vi "Multiple ToFs.vi"() -> ()   [LabVIEW 2014]
uses:
  <vilib>/Analysis/baseanly.llb/Mean (DBL).vi
  <vilib>/MakerHub/LINX/Public/Utilities/Open Local.vi
  <vilib>/MakerHub/LINX/LMH-LINX.lvlib
  <vilib>/Analysis/NI_AALBase.lvlib
panel:
  out "Sensor Error Code":u8
  out "Attempts":i32
  out "ToF 4":u8(slide) scale=0.0..80.0
  out "ToF 3":u8(slide) scale=0.0..80.0
  out "ToF 2":u8(slide) scale=0.0..80.0
  out "ToF 1":u8(slide) scale=0.0..80.0
  out "error out":errorcluster
  in  "Speed Read":bool
  out "Loop Rate (Hz)":u32
  out "range":dbl
  out "Array":dbl[](array[numeric])
  out "min value":dbl
  out "max value":dbl
  in  "Samples to Avg":i32=10
  in  "milliseconds to wait":u32=20
  in  "Stop":bool
  out "Distance":cluster{"Distance (mm)":u8, u8}(graph)
  # "0 = No error\n6 = early convergence estimate check failed\n7 = max convergence issue"
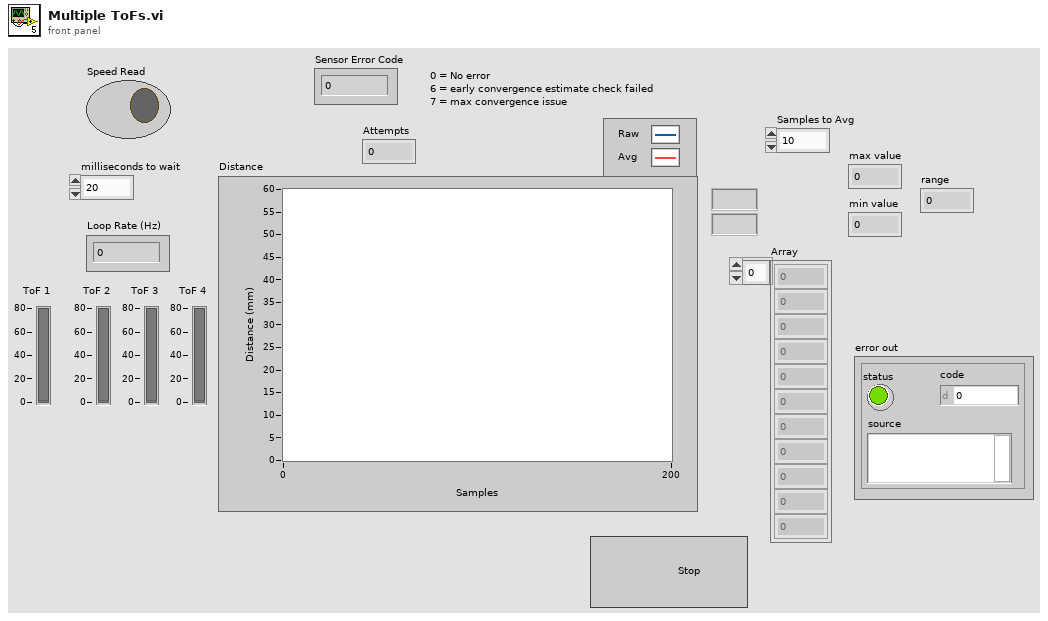
[diagram p1: front panel]
types:
  T1 = typedef "LMH-LINX.lvlib/LINX Ref.ctl" = cluster{"IO":T2, "Interface":T3, "LINX Device Config":T4}
  T2 = typedef "LMH-LINX.lvlib/Platform.ctl" = enum16{"Remote", "Local"}
  T3 = typedef "LMH-LINX.lvlib/Interface.ctl" = enum16{"Serial", "TCP"}
  T4 = typedef "LMH-LINX.lvlib/Device.lvlib/LINX Device Config.ctl" = cluster{"Interface":T3, "COM Port":refnum<visa-resource-name>, "TCP Configuration":T5, "Device Family":u8, "Device ID":u8, "Device Name":string, "TCP Ref":refnum<k5>, "Channels":T6}
  T5 = typedef "LMH-LINX.lvlib/Device.lvlib/TCP Config.ctl" = cluster{"IP Address":string, "Port":u16}
  T6 = typedef "LMH-LINX.lvlib/Channels.ctl" = cluster{"DI":u8[], "DO":u8[], "AI":u8[], "AO":u8[], "PWM":u8[], "QE":u8[], "UART":u8[], "I2C 2":u8[], "SPI":u8[], "CAN":u8[], "Servo":u8[], "AI Ref (V)":dbl, "AI Resolution (Bits)":u8, "AO Ref (V)":dbl, "AO Resolution (Bits)":u8}
  T7 = typedef "VL6180 Resource.ctl" = cluster{"I2C Channel":u8, "I2C Slave Address":u8}
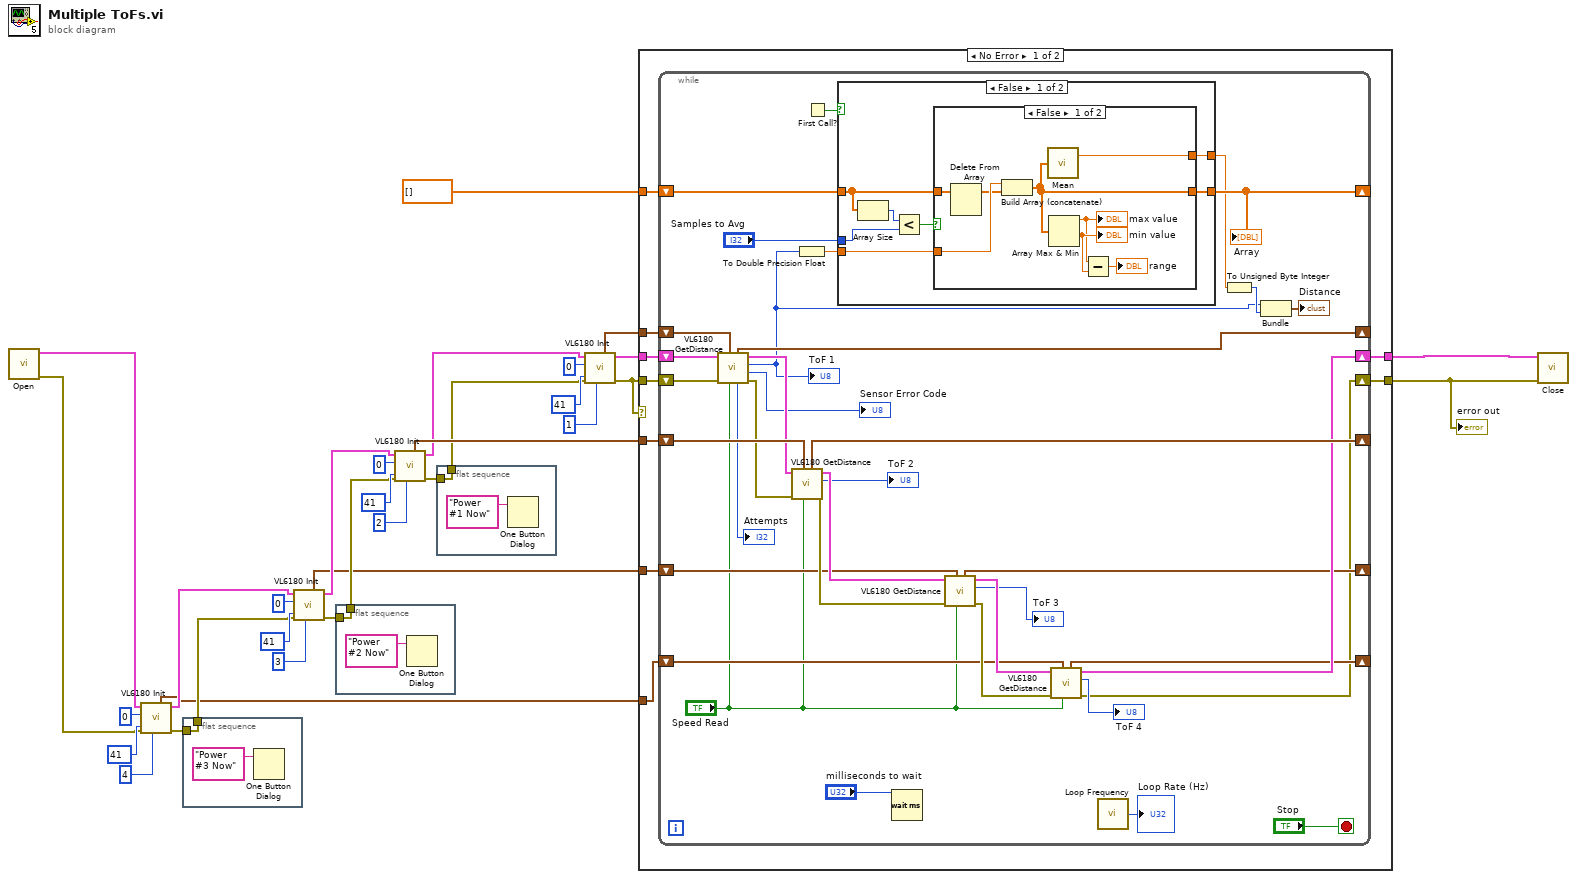
[diagram p0: block diagram]
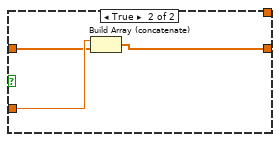
[diagram p2: hidden frame]
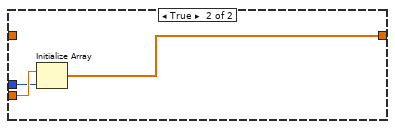
[diagram p3: hidden frame]
diagram:
  n1 = call-poly <vilib>:"Open.vi"() -> ("Error Out"=w1:errorcluster, "LINX Resource"=w2:T1)  [unwired: 9 in, 1 out]
  n2 = call "VL6180 Init.vi"("Change Slave Address"=u8 4, "Error In"=w1, "I2C Slave Address (0)"=u8 41, "I2C Channel"=u8 0, "LINX Resource"=w2) -> ("Error Out"=w10:errorcluster, "LINX Resource"=w5:T1, "VL6180 Resource"=w3:T7)  [unwired: 4 in]
  n3 = flat-sequence {
    tunnel: w10 -> [w33]
    tunnel: [w33] -> w6
    frame #0 {
      n4 = One Button Dialog(message="Power #3 Now") -> ()  [unwired: 1 in, 1 out]
    }
  }
  n5 = call "VL6180 Init.vi"("Change Slave Address"=u8 3, "Error In"=w6, "I2C Slave Address (0)"=u8 41, "I2C Channel"=u8 0, "LINX Resource"=w5) -> ("Error Out"=w17:errorcluster, "LINX Resource"=w8:T1, "VL6180 Resource"=w4:T7)  [unwired: 4 in]
  n6 = flat-sequence {
    tunnel: w17 -> [w35]
    tunnel: [w35] -> w7
    frame #0 {
      n7 = One Button Dialog(message="Power #2 Now") -> ()  [unwired: 1 in, 1 out]
    }
  }
  n8 = call "VL6180 Init.vi"("Change Slave Address"=u8 2, "Error In"=w7, "I2C Slave Address (0)"=u8 41, "I2C Channel"=u8 0, "LINX Resource"=w8) -> ("Error Out"=w20:errorcluster, "LINX Resource"=w9:T1, "VL6180 Resource"=w21:T7)  [unwired: 4 in]
  n9 = flat-sequence {
    tunnel: w20 -> [w37]
    tunnel: [w37] -> w19
    frame #0 {
      n10 = One Button Dialog(message="Power #1 Now") -> ()  [unwired: 1 in, 1 out]
    }
  }
  n11 = call "VL6180 Init.vi"("Change Slave Address"=u8 1, "Error In"=w19, "I2C Slave Address (0)"=u8 41, "I2C Channel"=u8 0, "LINX Resource"=w9) -> ("Error Out"=w28:errorcluster, "LINX Resource"=w29:T1, "VL6180 Resource"=w27:T7)  [unwired: 4 in]
  n12 = case shown="No Error" w28 {
    tunnel: w28 -> [w47 w105]
    tunnel: [w46 w105] -> w18
    tunnel: [w45 w106] -> w26
    tunnel: dbl[] [] -> [w44 _]
    tunnel: w29 -> [w43 w106]
    tunnel: w27 -> [w42 _]
    tunnel: w21 -> [w41 _]
    tunnel: w4 -> [w40 _]
    tunnel: w3 -> [w39 _]
    frame No Error {
      n13 = while {
        shift-right: [w62] -> w45
        shift-left: w43 -> [w72]
        shift-right: [w50] -> w46
        shift-left: w47 -> [w71]
        shift-right: [w78] -> _
        shift-left: w44 -> [w77]
        shift-right: [w69] -> _
        shift-left: w42 -> [w70]
        shift-right: [w65] -> _
        shift-left: w41 -> [w68]
        shift-right: [w58] -> _
        shift-left: w40 -> [w59]
        shift-right: [w57] -> _
        shift-left: w39 -> [w56]
        stop <- "Stop" stop-if-true
        n14 = call "VL6180 GetDistance.vi"("Speed Read"="Speed Read", "VL6180 Resource in"=w70, "error in (no error)"=w71, "LINX Resource"=w72) -> ("error out"=w66:errorcluster, "Sensor Error Code"=→"Sensor Error Code":u8, "Distance (mm)"=w52:u8, "LINX Resource"=w67:T1, "Attempts"=→"Attempts":i32, "VL6180 Resource out"=w69:T7)  [unwired: 2 in]
        "ToF 1" <- w52
        n15 = call "VL6180 GetDistance.vi"("Speed Read"="Speed Read", "VL6180 Resource in"=w68, "error in (no error)"=w66, "LINX Resource"=w67) -> ("error out"=w61:errorcluster, "Distance (mm)"=→"ToF 2":u8, "LINX Resource"=w64:T1, "VL6180 Resource out"=w65:T7)  [unwired: 2 in, 2 out]
        n16 = To Double Precision Float(number=w52) -> (double precision float=w80:dbl)
        n17 = First Call?() -> (First Call?: T/F=w81:bool)
        n18 = case shown="False" w81 {
          tunnel: w80 -> [w87 w104]
          tunnel: "Samples to Avg" -> [w88 w103]
          tunnel: [w85 w102] -> w78
          tunnel: w77 -> [w86 _]
          tunnel: [w84 _] -> w74
          frame False {
            n19 = Array Size(array=w86) -> (size(s)=w89:i32)
            n20 = Less?(x=w89, y=w88) -> (x < y?=w90:bool)
            n21 = case shown="False" w90 {
              tunnel: w87 -> [w97 w101]
              tunnel: w86 -> [w98 w100]
              tunnel: [w95 w99] -> w85
              tunnel: [w91 _] -> w84
              frame False {
                n22 = Delete From Array(array=w98) -> (array with subset deleted=w96:dbl[])  [unwired: 2 in, 1 out]
                n23 = Build Array (concatenate)(w97, w96) -> (w95:dbl[])
                n24 = call-poly <vilib>:"Mean.vi"("X"=w95) -> ("mean"=w91:dbl)  [unwired: 1 out]
                n25 = Array Max & Min(array=w95) -> (max value=w93:dbl, min value=w94:dbl)  [unwired: 2 out]
                "max value" <- w93
                "min value" <- w94
                n26 = Subtract(x=w93, y=w94) -> (x-y=→"range":dbl)
              }
              frame True {
                n27 = Build Array (concatenate)(w101, w100) -> (w99:dbl[])
              }
            }
          }
          frame True {
            n28 = Initialize Array(w104, w103) -> (w102:dbl[])
          }
        }
        "Array" <- w78
        n29 = Wait (ms)(milliseconds to wait="milliseconds to wait") -> ()  [unwired: 1 out]
        n30 = call "VL6180 GetDistance.vi"("Speed Read"="Speed Read", "VL6180 Resource in"=w59, "error in (no error)"=w61, "LINX Resource"=w64) -> ("error out"=w60:errorcluster, "Distance (mm)"=→"ToF 3":u8, "LINX Resource"=w63:T1, "VL6180 Resource out"=w58:T7)  [unwired: 2 in, 2 out]
        n31 = call "VL6180 GetDistance.vi"("Speed Read"="Speed Read", "VL6180 Resource in"=w56, "error in (no error)"=w60, "LINX Resource"=w63) -> ("error out"=w50:errorcluster, "Distance (mm)"=→"ToF 4":u8, "LINX Resource"=w62:T1, "VL6180 Resource out"=w57:T7)  [unwired: 2 in, 2 out]
        n32 = call <vilib>:"Loop Frequency.vi"() -> ("Loop Rate (Hz)"=→"Loop Rate (Hz)":u32)
        n33 = To Unsigned Byte Integer(number=w74) -> (unsigned 8bit integer=w73:u8)
        n34 = Bundle("Distance (mm)"=w52, w73) -> (→"Distance":cluster{"Distance (mm)":u8, u8})  [unwired: 1 in]
      }
    }
    frame Error {
    }
  }
  "error out" <- w18
  n35 = call <vilib>:"Close.vi"("Error In"=w18, "LINX Resource"=w26) -> ()  [unwired: 9 in, 1 out]
